vi "Test Serialize Waveforms.vi"(8 "error in (no error)":errorcluster) -> (0 "error out":errorcluster)   [LabVIEW 2013]
uses:
  src/Serializer/JSON Serializer/JSON Serializer.lvclass
  <vilib>/addons/_JKI Toolkits/Caraya/classes/Test/Test.lvclass
  <vilib>/addons/_JKI Toolkits/Caraya/classes/Assert/Assert.lvclass
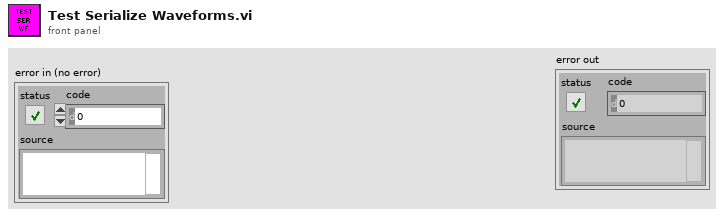
[diagram p1: front panel]
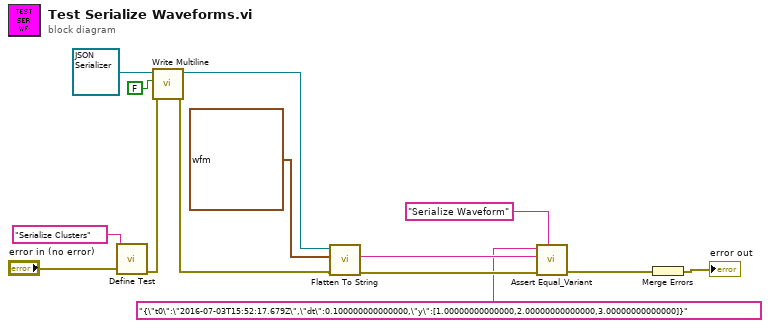
[diagram p0: block diagram]
diagram:
  n1 = call <vilib>:"Define Test.vi"("error in (no error)"="error in (no error)", "Label (VI Title)"="Serialize Clusters") -> ("error out"=w10:errorcluster)  [unwired: 9 in]
  n2 = call-dynamic "Write Multiline.vi"("error in (no error)"=w10, "Multiline"=FALSE, "JSON Serializer in"=refnum<class "JSON Serializer.lvclass"> refnum ("JKI JSON Serialization.lvlib:JSON Serializer.lvclass")) -> ("error out"=w4:errorcluster, "JSON Serializer out"=w3:refnum<class "JSON Serializer.lvclass">)  [unwired: 7 in]
  n3 = call-dynamic "Flatten To String.vi"("error in (no error)"=w4, "Variant"=waveform(dbl) {"t0"=timestamp(3550405937.679 s since 1904-01-01), "dt"=0.1, "Y"=[1.0, 2.0, 3.0]} ("Waveform"), "JSON Serializer in"=w3) -> ("error out"=w7:errorcluster, "String"=w6:string)  [unwired: 6 in, 1 out]
  n4 = call <vilib>:"Assert Equal_Variant.vi"("Label"="Serialize Waveform", "error in (no error)"=w7, "Y"=w6, "X"="{\"t0\":\"2016-07-03T15:52:17.679Z\",\"dt\":0.100000000000000,\"y\":[1.00000000000000,2.00000000000000,3.00000000000000]}") -> ("error out"=w5:errorcluster)  [unwired: 7 in]
  n5 = Merge Errors(w5) -> (→"error out":errorcluster)
